vi "power_supply_server_2.vi"(10 "power_supply 3&4":refnum<visa-resource-name>, 11 "power_supply2 load":bool) -> ()   [LabVIEW 2020]
uses:
  status/stop software.vi
  status/emergency stop.vi
  status/pause3.vi
  status/pause4.vi
  <instrlib>/GPD-3303/GPD-3303.lvlib
panel:
  out "pause4?":bool
  out "pause3?":bool
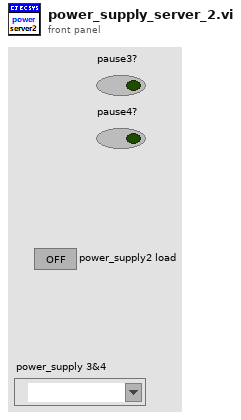
[diagram p1: front panel]
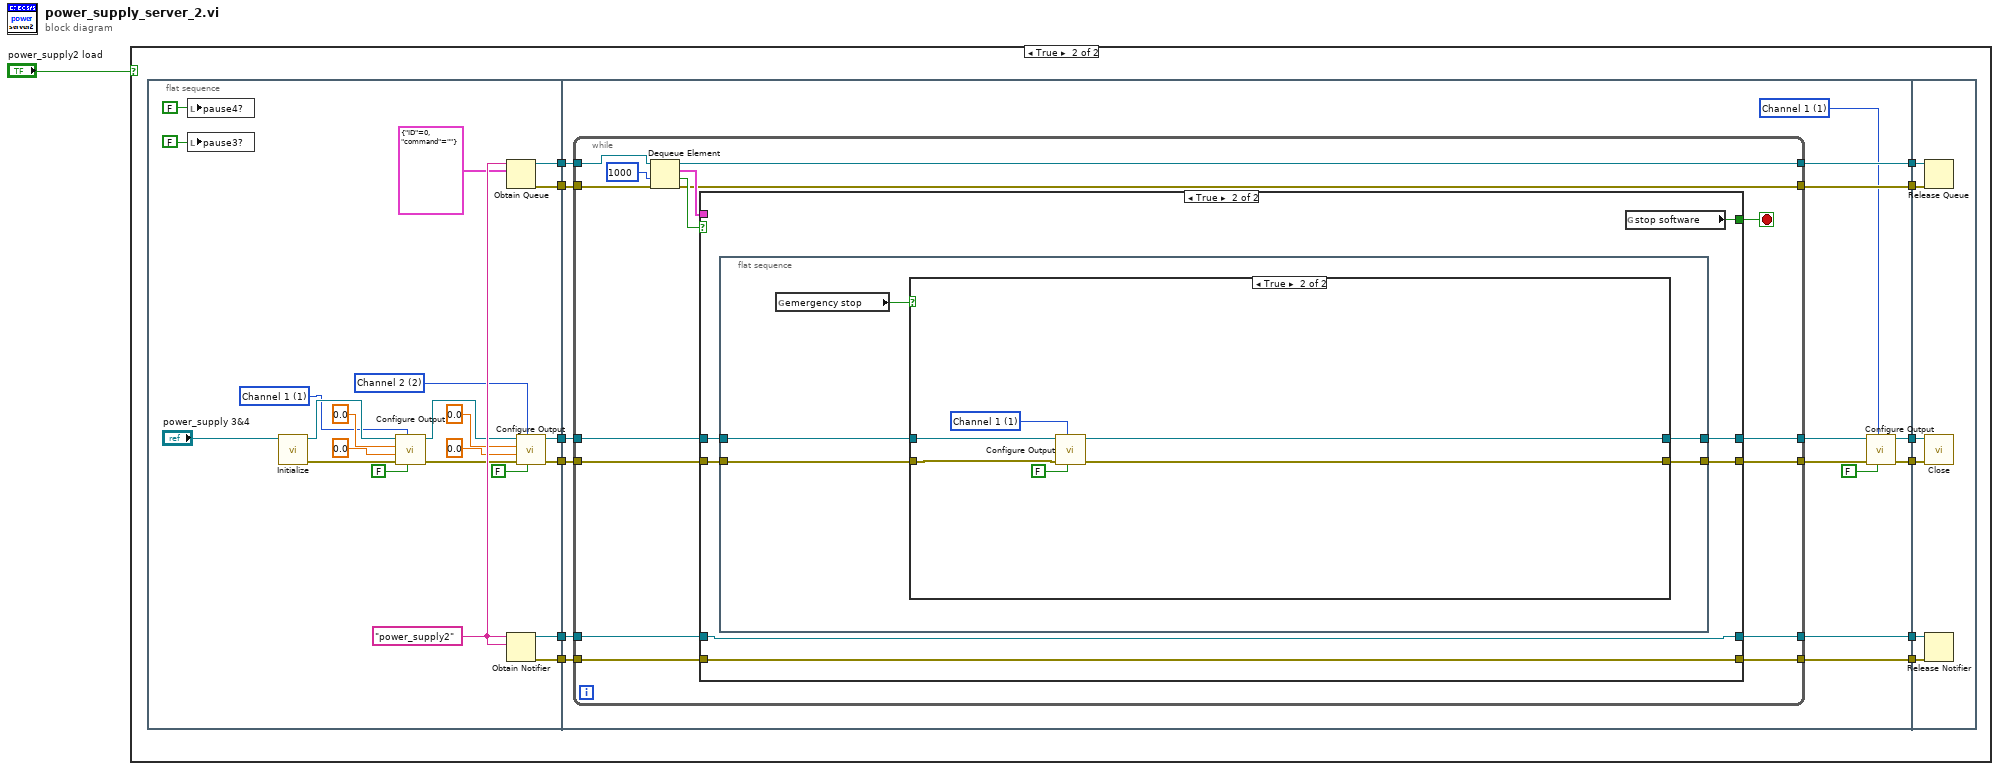
[diagram p0: block diagram]
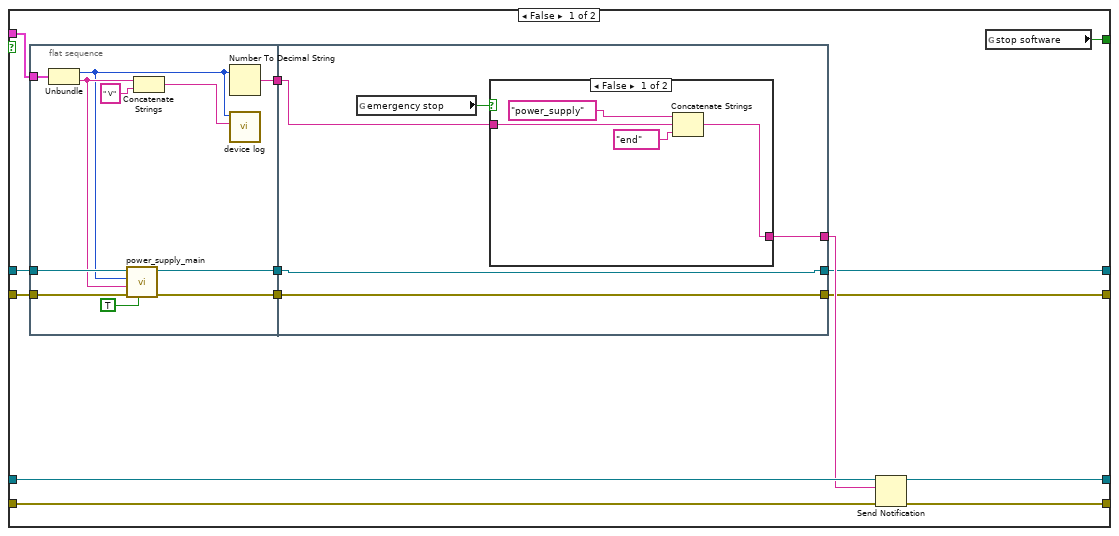
[diagram p3: hidden frame]
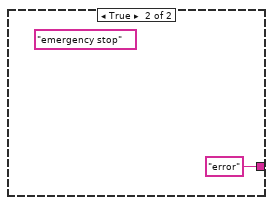
[diagram p4: hidden frame]
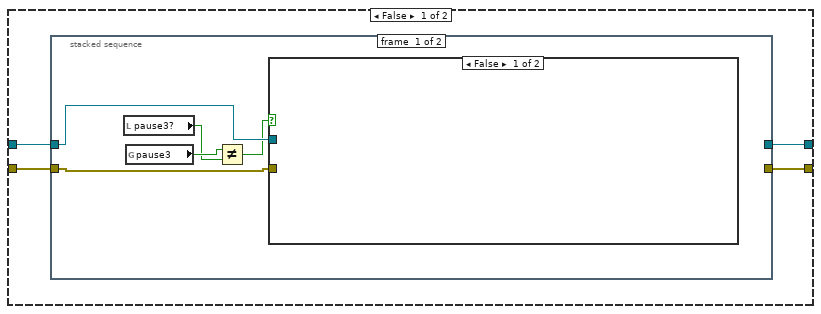
[diagram p5: hidden frame]
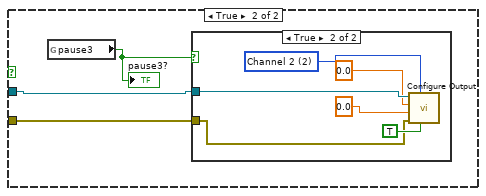
[diagram p6: hidden frame]
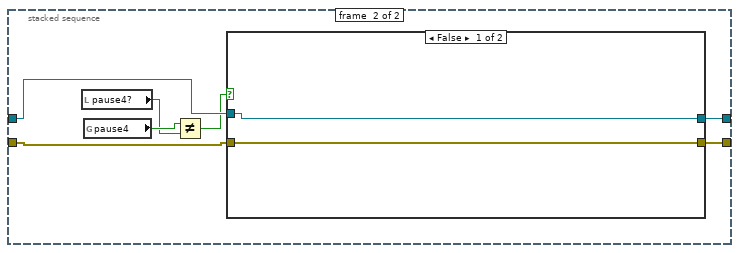
[diagram p8: hidden frame]
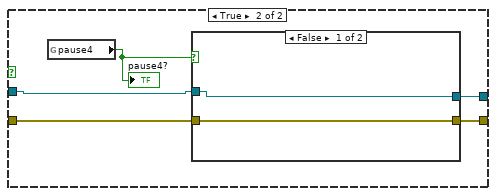
[diagram p9: hidden frame]
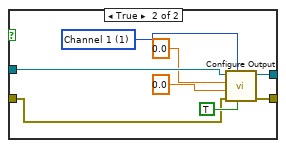
[diagram p10: hidden frame]
diagram:
  n1 = case shown="True" "power_supply2 load" {
    frame False {
    }
    frame True {
      n2 = flat-sequence {
        tunnel: [w32] -> w13
        tunnel: [w36] -> w12
        tunnel: [w35] -> w11
        tunnel: [w34] -> w10
        tunnel: [w19] -> w5
        tunnel: [w18] -> w4
        tunnel: w13 -> [w52]
        tunnel: w12 -> [w51]
        tunnel: w11 -> [w50]
        tunnel: w10 -> [w49]
        tunnel: [w48] -> w9
        tunnel: [w47] -> w8
        tunnel: [w46] -> w7
        tunnel: [w45] -> w6
        tunnel: w5 -> [w44]
        tunnel: w4 -> [w43]
        tunnel: [w38] -> w3
        tunnel: [w37] -> w2
        tunnel: w9 -> [w169]
        tunnel: w8 -> [w168]
        tunnel: w7 -> [w167]
        tunnel: w6 -> [w166]
        tunnel: w3 -> [w165]
        tunnel: w2 -> [w164]
        frame #0 {
          w16 = 2 items=["Channel 1"=1, "Channel 2"=2] ("Channel (1: Channel 1)")
          w17 = 1 items=["Channel 1"=1, "Channel 2"=2] ("Channel (1: Channel 1)")
          w33 = "power_supply2" ("name (unnamed)")
          n3 = local write "pause4?"(FALSE ("pause4?")) -> ()
          n4 = local write "pause3?"(FALSE ("pause3?")) -> ()
          n5 = call <instrlib>:"Initialize.vi"("VISA resource name"="power_supply 3&4") -> ("error out"=w30:errorcluster, "VISA resource name out"=w29:refnum<visa-resource-name>)  [unwired: 9 in]
          n6 = call <instrlib>:"Configure Output.vi"("Enable Output (T: Enable)"=FALSE, "Channel (1: Channel 1)"=w17, "error in (no error)"=w30, "Current Level (0.0 V)"=0.0, "Voltage Level (0.0 V)"=0.0, "VISA resource name"=w29) -> ("error out"=w28:errorcluster, "VISA resource name out"=w27:refnum<visa-resource-name>)  [unwired: 4 in]
          n7 = Obtain Queue(name (unnamed)=w33, element data type=cluster{"ID":u8, "command":string} {"ID"=0, "command"=""} ("参数")) -> (queue out=w32:refnum<queue>, error out=w36:errorcluster)  [unwired: 3 in, 1 out]
          n8 = Obtain Notifier(name (unnamed)=w33, notification data type=w33) -> (notifier out=w35:refnum<notifier>, error out=w34:errorcluster)  [unwired: 2 in, 1 out]
          n9 = call <instrlib>:"Configure Output.vi"("Enable Output (T: Enable)"=FALSE, "Channel (1: Channel 1)"=w16, "error in (no error)"=w28, "Current Level (0.0 V)"=0.0, "Voltage Level (0.0 V)"=0.0, "VISA resource name"=w27) -> ("error out"=w18:errorcluster, "VISA resource name out"=w19:refnum<visa-resource-name>)  [unwired: 4 in]
        }
        frame #1 {
          w41 = 1 items=["Channel 1"=1, "Channel 2"=2] ("Channel (1: Channel 1)")
          n10 = while {
            tunnel: w52 -> [w67]
            tunnel: w51 -> [w66]
            tunnel: w50 -> [w62]
            tunnel: w49 -> [w61]
            tunnel: [w60] -> w48
            tunnel: [w59] -> w47
            tunnel: [w58] -> w46
            tunnel: [w57] -> w45
            tunnel: w44 -> [w56]
            tunnel: w43 -> [w55]
            tunnel: [w54] -> w40
            tunnel: [w53] -> w39
            stop <- w64 stop-if-true
            n11 = Dequeue Element(queue=w67, timeout in ms (-1)=1000, error in (no error)=w66) -> (queue out=w58:refnum<queue>, element=w63:cluster{"ID":u8, "command":string}, timed out?=w65:bool, error out=w57:errorcluster)
            n12 = case shown="True" w65 {
              tunnel: [w78 w108] -> w64
              tunnel: w63 -> [w74 _]
              tunnel: w62 -> [w82 w110]
              tunnel: w61 -> [w81 w109]
              tunnel: [w80 w110] -> w60
              tunnel: [w79 w109] -> w59
              tunnel: w56 -> [w72 w107]
              tunnel: w55 -> [w71 w106]
              tunnel: [w70 w105] -> w54
              tunnel: [w69 w104] -> w53
              frame False {
                n13 = flat-sequence {
                  tunnel: w74 -> [w93]
                  tunnel: [w92] -> w77
                  tunnel: w72 -> [w89]
                  tunnel: [w86] -> w76
                  tunnel: [w85] -> w75
                  tunnel: w71 -> [w83]
                  tunnel: w77 -> [w97]
                  tunnel: [w96] -> w73
                  tunnel: w76 -> [w95]
                  tunnel: [w95] -> w70
                  tunnel: [w94] -> w69
                  tunnel: w75 -> [w94]
                  frame #0 {
                    n14 = Unbundle(w93) -> ("ID"=w87:u8, "command"=w88:string)
                    n15 = call "power_supply_main.vi"("Enable Output (T: Enable)"=TRUE, "error in (no error)"=w83, "command"=w88, "channel"=w87, "VISA resource name"=w89) -> ("error out"=w85:errorcluster, "VISA resource name out"=w86:refnum<visa-resource-name>)  [unwired: 5 in]
                    n16 = Concatenate Strings(w88, " V" ("command")) -> (w91:string)
                    n17 = Number To Decimal String(number=w87) -> (decimal integer string=w92:string)  [unwired: 1 in]
                    n18 = call "device log.vi"("new element/subarray"=w91, "worker ID"=w87) -> ()  [unwired: 10 in]
                  }
                  frame #1 {
                    n19 = global read "emergency stop.vi" "emergency stop"() -> (w98:bool)
                    n20 = case shown="False" w98 {
                      tunnel: [w100 "error" ("notification")] -> w96
                      tunnel: w97 -> [w99 _]
                      frame False {
                        n21 = Concatenate Strings("power_supply" ("string"), w99, "end" ("notification")) -> (w100:string)
                      }
                      frame True {
                        (unwired) "emergency stop" ("power_supply_1 status")
                      }
                    }
                  }
                }
                n22 = Send Notification(notification=w73, notifier=w82, error in (no error)=w81) -> (notifier out=w80:refnum<notifier>, error out=w79:errorcluster)
                n23 = global read "stop software.vi" "stop software"() -> (w78:bool)
              }
              frame True {
                n24 = flat-sequence {
                  tunnel: w107 -> [w114]
                  tunnel: w106 -> [w113]
                  tunnel: [w112] -> w105
                  tunnel: [w111] -> w104
                  frame #0 {
                    n25 = global read "emergency stop.vi" "emergency stop"() -> (w115:bool)
                    n26 = case shown="True" w115 {
                      tunnel: w114 -> [w119 w161]
                      tunnel: w113 -> [w118 w160]
                      tunnel: [w117 w159] -> w112
                      tunnel: [w116 w158] -> w111
                      frame False {
                        n27 = stacked-sequence {
                          tunnel: w119 -> [w124 w140]
                          tunnel: w118 -> [w123 w139]
                          tunnel: [_ w138] -> w117
                          tunnel: [_ w137] -> w116
                          frame #0 {
                            n28 = local read "pause3?"() -> (w121:bool)
                            n29 = global read "pause3.vi" "pause3"() -> (w122:bool)
                            n30 = Not Equal?(x=w122, y=w121) -> (x != y?=w120:bool)
                            n31 = case shown="False" w120 {
                              tunnel: w124 -> [_ w127]
                              tunnel: w123 -> [_ w126]
                              frame False {
                              }
                              frame True {
                                n32 = global read "pause3.vi" "pause3"() -> (w125:bool)
                                "pause3?" <- w125
                                n33 = case shown="True" w125 {
                                tunnel: w127 -> [_ w131]
                                tunnel: w126 -> [_ w130]
                                frame False {
                                }
                                frame True {
                                w132 = 2 items=["Channel 1"=1, "Channel 2"=2] ("Channel (1: Channel 1)")
                                n34 = call <instrlib>:"Configure Output.vi"("Enable Output (T: Enable)"=TRUE, "Channel (1: Channel 1)"=w132, "error in (no error)"=w130, "Current Level (0.0 V)"=0.0, "Voltage Level (0.0 V)"=0.0, "VISA resource name"=w131) -> ()  [unwired: 4 in, 2 out]
                                }
                                }
                              }
                            }
                          }
                          frame #1 {
                            n35 = local read "pause4?"() -> (w134:bool)
                            n36 = global read "pause4.vi" "pause4"() -> (w135:bool)
                            n37 = Not Equal?(x=w135, y=w134) -> (x != y?=w136:bool)
                            n38 = case shown="False" w136 {
                              tunnel: w140 -> [w142 w147]
                              tunnel: w139 -> [w141 w146]
                              tunnel: [w142 w145] -> w138
                              tunnel: [w141 w144] -> w137
                              frame False {
                              }
                              frame True {
                                n39 = global read "pause4.vi" "pause4"() -> (w143:bool)
                                "pause4?" <- w143
                                n40 = case shown="False" w143 {
                                tunnel: w147 -> [w149 w155]
                                tunnel: [w149 w153] -> w145
                                tunnel: w146 -> [w148 w154]
                                tunnel: [w148 w152] -> w144
                                frame False {
                                }
                                frame True {
                                w156 = 1 items=["Channel 1"=1, "Channel 2"=2] ("Channel (1: Channel 1)")
                                n41 = call <instrlib>:"Configure Output.vi"("Enable Output (T: Enable)"=TRUE, "Channel (1: Channel 1)"=w156, "error in (no error)"=w154, "Current Level (0.0 V)"=0.0, "Voltage Level (0.0 V)"=0.0, "VISA resource name"=w155) -> ("error out"=w152:errorcluster, "VISA resource name out"=w153:refnum<visa-resource-name>)  [unwired: 4 in]
                                }
                                }
                              }
                            }
                          }
                        }
                      }
                      frame True {
                        w162 = 1 items=["Channel 1"=1, "Channel 2"=2] ("Channel (1: Channel 1)")
                        n42 = call <instrlib>:"Configure Output.vi"("Enable Output (T: Enable)"=FALSE, "Channel (1: Channel 1)"=w162, "error in (no error)"=w160, "VISA resource name"=w161) -> ("error out"=w158:errorcluster, "VISA resource name out"=w159:refnum<visa-resource-name>)  [unwired: 6 in]
                      }
                    }
                  }
                }
                n43 = global read "stop software.vi" "stop software"() -> (w108:bool)
              }
            }
          }
          n44 = call <instrlib>:"Configure Output.vi"("Enable Output (T: Enable)"=FALSE, "Channel (1: Channel 1)"=w41, "error in (no error)"=w39, "VISA resource name"=w40) -> ("error out"=w38:errorcluster, "VISA resource name out"=w37:refnum<visa-resource-name>)  [unwired: 6 in]
        }
        frame #2 {
          n45 = Release Queue(queue=w167, error in (no error)=w166) -> ()  [unwired: 1 in, 3 out]
          n46 = call <instrlib>:"Close.vi"("error in (no error)"=w165, "VISA resource name"=w164) -> ()  [unwired: 9 in, 1 out]
          n47 = Release Notifier(notifier=w169, error in (no error)=w168) -> ()  [unwired: 1 in, 3 out]
        }
      }
    }
  }
